vi "Min_Value.vi"() -> ()   [LabVIEW 2024]
panel:
  out "Array":dbl[](array[numeric])
  out "min value":dbl
  out "min index(es)":i32
  in  "Numeric":i32
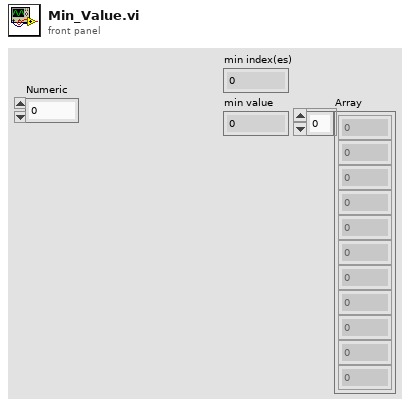
[diagram p1: front panel]
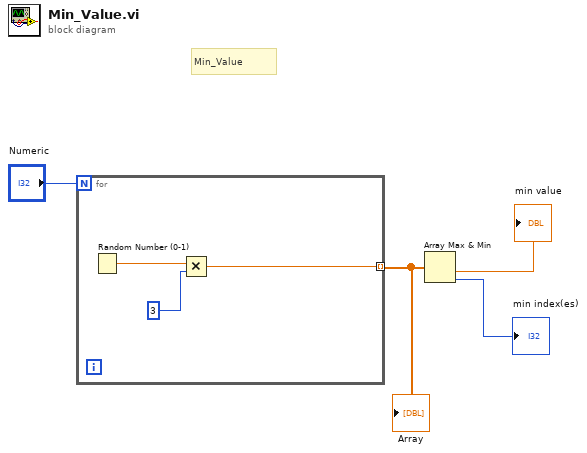
[diagram p0: block diagram]
diagram:
  # "Min_Value"
  n1 = for {
    N: "Numeric" -> [_]
    tunnel: [w5] -> w3 mode=indexing
    n2 = Random Number (0-1)() -> (number: 0 to 1=w7:dbl)
    n3 = Multiply(x=w7, y=3) -> (x*y=w5:dbl)
  }
  "Array" <- w3
  n4 = Array Max & Min(array=w3) -> (min value=→"min value":dbl, min index (indices)=→"min index(es)":i32)  [unwired: 2 out]
